vi "Autonomous Independent.vi"() -> ()   [LabVIEW 2013]
doc: "This VI is called when autonomous begins, and will automatically be terminated when autonomous ends. You can carry out timed or sensor driven robot movement independently without needing to return to the caller."
uses:
  Robot Global Data.vi
  <vilib>/Rock Robotics/WPI/Solenoid/Deprecated/WPI_SolenoidSetBool.vi
  <vilib>/Rock Robotics/WPI/Compressor/WPI_CompressorGetSetRefNum.vi
  <vilib>/Rock Robotics/WPI/RobotDrive/WPI_RobotDriveArcadeDrive_Standard(NoSaturation).vi
panel:
  in  "1 Ball Standard Auton Drive Length 2":dbl=11.0
  in  "final pickup delay":u32=1250
  in  "reload timeout 2":u32=4500
  in  "adjust out delay":u32=500
  in  "2 ball auton drive length":dbl=14.2
  in  "1st pickup delay 2":u32=500
  in  "Driving Shot Distance":dbl=10.0
  in  "Driving Shoot total distance":dbl=14.0
  in  "1 Ball Standard Auton Drive Length":dbl=11.0
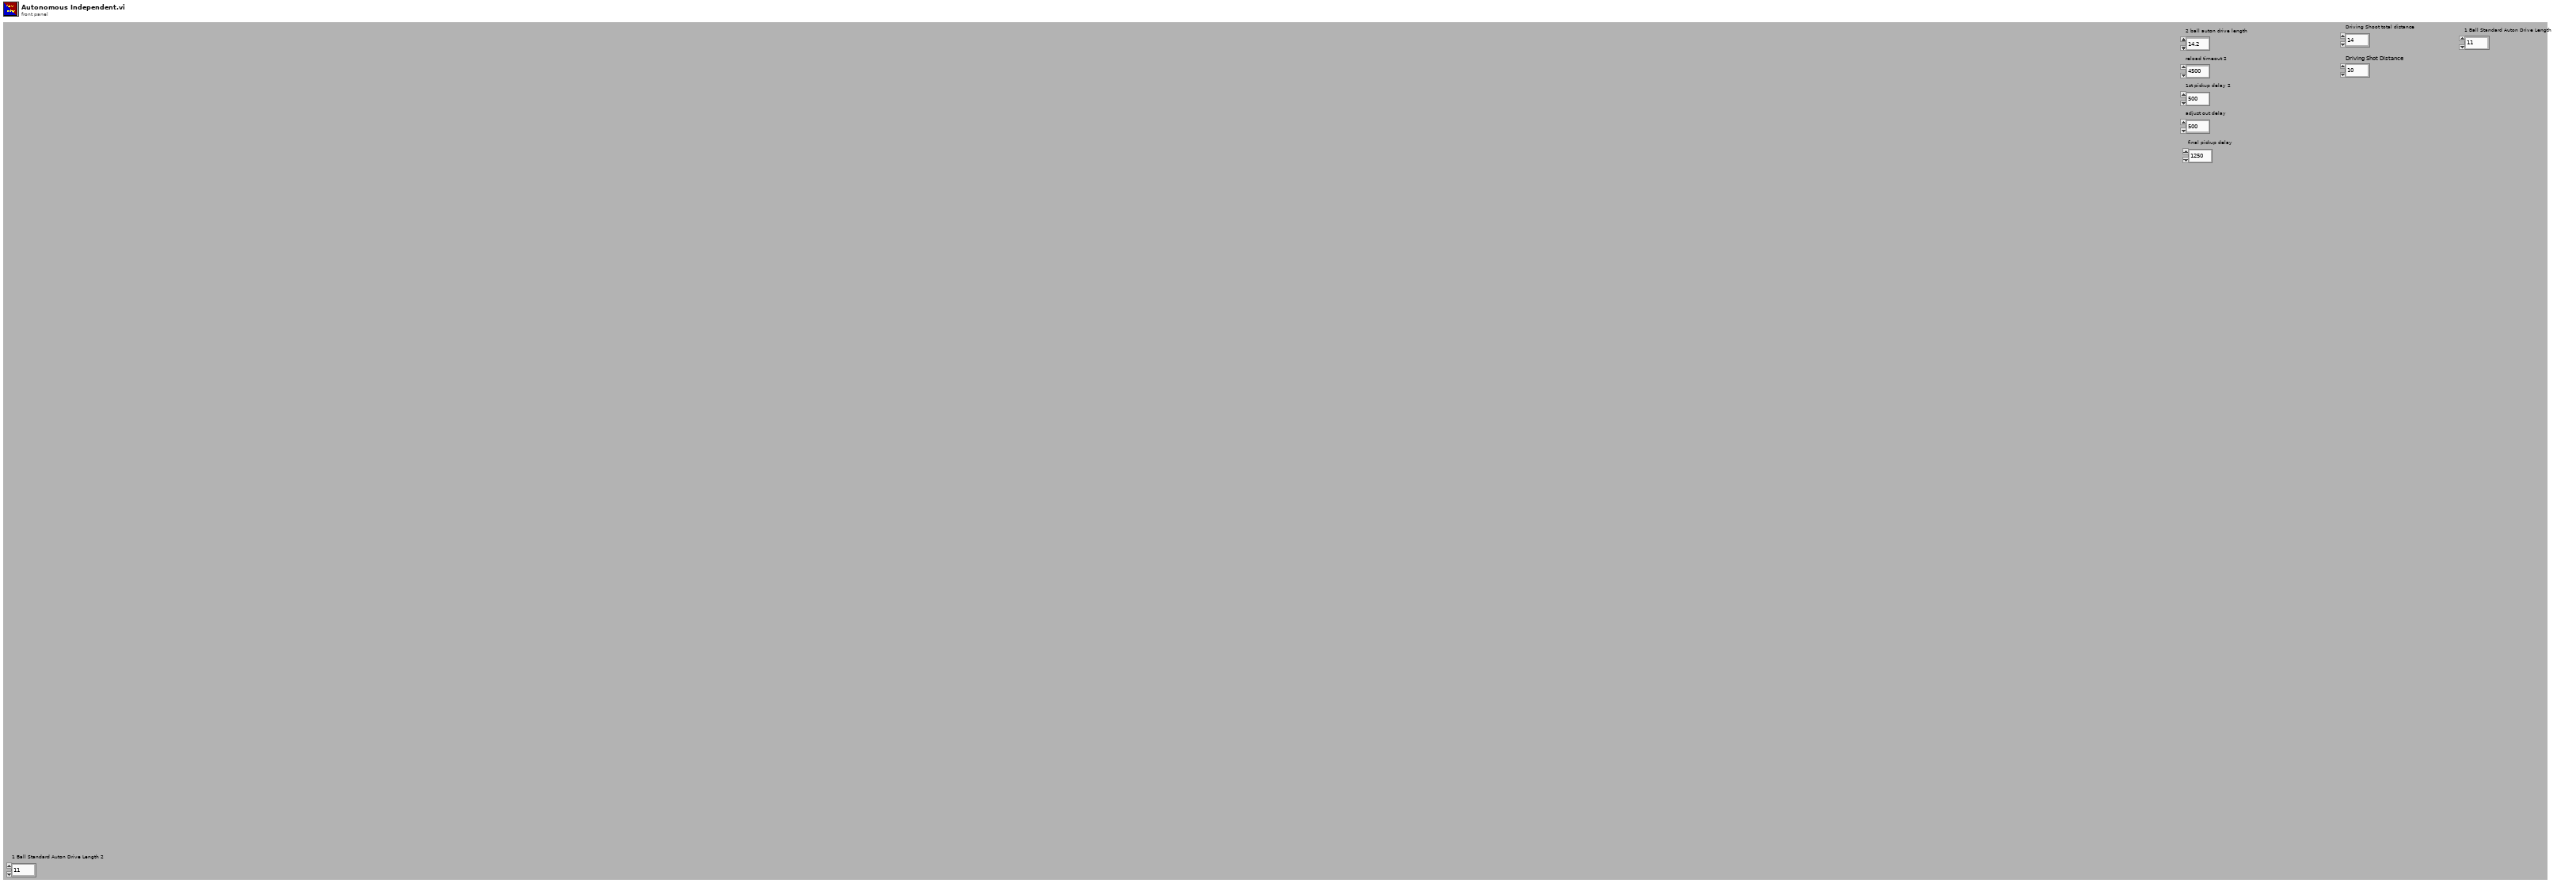
[diagram p1: front panel]
types:
  T1 = typedef "WPI_CompressorDevRef.ctl" = cluster{"DevStatus":errorcluster, "DigitalInputDevRef":T2, "RelayDevRef":T5}
  T2 = typedef "WPI_DigitalInputDevRef.ctl" = cluster{"DevStatus":errorcluster, "DIO Channel":T3, "Digital Module":T4}
  T3 = typedef "FPGA_DIOChannel.ctl" = enum8{"DIO 1", "DIO 2", "DIO 3", "DIO 4", "DIO 5", "DIO 6", "DIO 7", "DIO 8", "DIO 9", "DIO 10", "DIO 11", "DIO 12", "DIO 13", "DIO 14", "Invalid"}
  T4 = typedef "FPGA_TypedefDigitalModule.ctl" = enum16{"Digital Module 1", "Digital Module 2"}
  T5 = typedef "WPI_RelayDevRef.ctl" = cluster{"DevStatus":errorcluster, "Relay Channel":T6, "Digital Module":T4, "Relay Direction":T7}
  T6 = typedef "FPGA_DIORelayChannel.ctl" = enum8{"Relay 1", "Relay 2", "Relay 3", "Relay 4", "Relay 5", "Relay 6", "Relay 7", "Relay 8", "Invalid"}
  T7 = typedef "WPI_RelayDirection.ctl" = enum16{"Both directions", "Forward only", "Reverse only"}
  T8 = typedef "WPI_EncoderDevRef.ctl" = cluster{"DevStatus":errorcluster, "EncoderIndex":T9, "CounterIndex":T10, "DistancePerCount":dbl, "Decoding Type":T11}
  T9 = typedef "FPGA_EncoderIdx.ctl" = enum8{"Enc 0", "Enc 1", "Enc 2", "Enc 3", "Invalid"}
  T10 = typedef "FPGA_CounterCtrSystemIndex.ctl" = enum8{"Ctr 0", "Ctr 1", "Ctr 2", "Ctr 3", "Ctr 4", "Ctr 5", "Ctr 6", "Ctr 7", "Invalid"}
  T11 = typedef "WPI_EncoderType.ctl" = enum16{"1x", "2x", "4x"}
  T12 = typedef "WPI_SolenoidDevRef.ctl" = cluster{"DevStatus":errorcluster, "Solenoid Module":T13, "Forward Solenoid Channel":T14, "Reverse Solenoid Channel":T14}
  T13 = typedef "FPGA_TypedefSolenoidModule.ctl" = enum16{"Solenoid Module 1", "Solenoid Module 2"}
  T14 = typedef "WPI_SolenoidChannel.ctl" = enum8{"Solenoid 1", "Solenoid 2", "Solenoid 3", "Solenoid 4", "Solenoid 5", "Solenoid 6", "Solenoid 7", "Solenoid 8", "Invalid"}
  T15 = typedef "WPI_GyroDevRef.ctl" = cluster{"DevStatus":errorcluster, "Analog Module":T16, "Analog Channel":T17, "Offset":dbl, "Gain (VoltsPerDegree/Second)":dbl}
  T16 = typedef "FPGA_TypedefAnalogModule.ctl" = enum16{"Analog Module 1", "Analog Module 2"}
  T17 = typedef "FPGA_AIChannel.ctl" = enum8{"AI 1", "AI 2", "AI 3", "AI 4", "AI 5", "AI 6", "AI 7", "AI 8", "Invalid"}
  T18 = typedef "WPI_MotorControlDeviceRef.ctl" = cluster{"DeviceStatus":errorcluster, "Type":enum16{"PWM", "CAN"}, "PWM":cluster{"Digital Module":T4, "PWM Channel":T19, "DeadBand":T20}, "CAN":cluster{"Device Number":u8, "Control Mode":T21, "Semaphore":T22, "Max Vout":dbl}, "Invert":bool, "TransformRef":T23, "InvTransformRef":T23}
  T19 = typedef "FPGA_DIOPWMChannel.ctl" = enum8{"PWM 1", "PWM 2", "PWM 3", "PWM 4", "PWM 5", "PWM 6", "PWM 7", "PWM 8", "PWM 9", "PWM 10", "Invalid"}
  T20 = typedef "WPI_PWMDeadband.ctl" = cluster{"Name":string, "maxPositivePwm":i32, "minPositivePwm":i32, "centerPwm":i32, "maxNegativePwm":i32, "minNegativePwm":i32, "angularRange":u16}
  T21 = typedef "WPI_CANJaguar_ControlMode.ctl" = enum8{"Percent VBus", "Current", "Speed", "Position", "Voltage"}
  T22 = typedef "Semaphore RefNum" = refnum<k1>
  T23 = typedef "WPI_PWMTransform_ConPane.ctl" = refnum<vi>
  T24 = typedef "WPI_AnalogChannelDevRef.ctl" = cluster{"DevStatus":errorcluster, "Analog Module":T16, "Analog Channel":T17}
  T25 = typedef "WPI_RobotDriveDevRef.ctl" = cluster{"DevStatus":errorcluster, "Motors[]":T18[], "Square Inputs":bool, "Max Output":dbl, "Isochronous":bool}
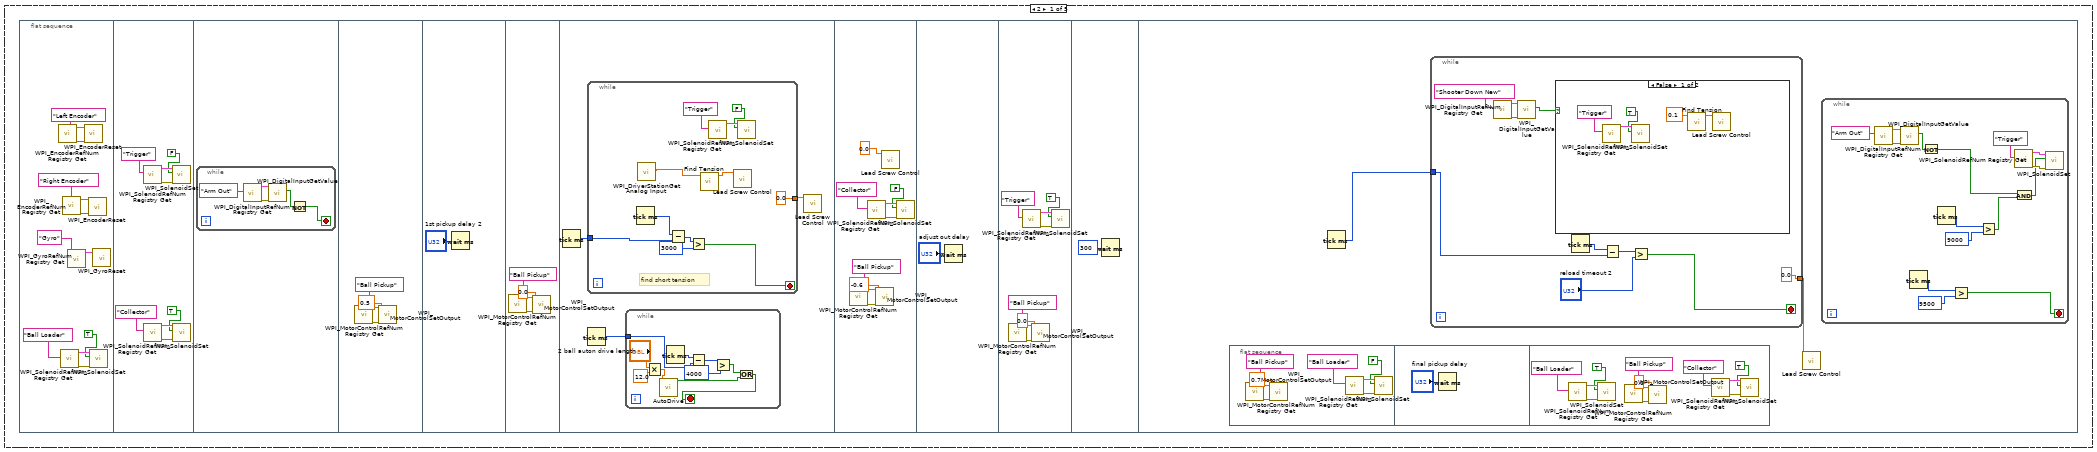
[diagram p2: hidden frame]
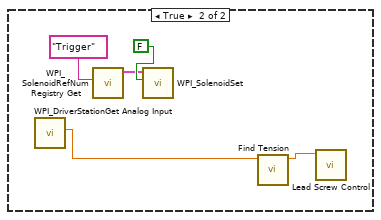
[diagram p3: hidden frame]
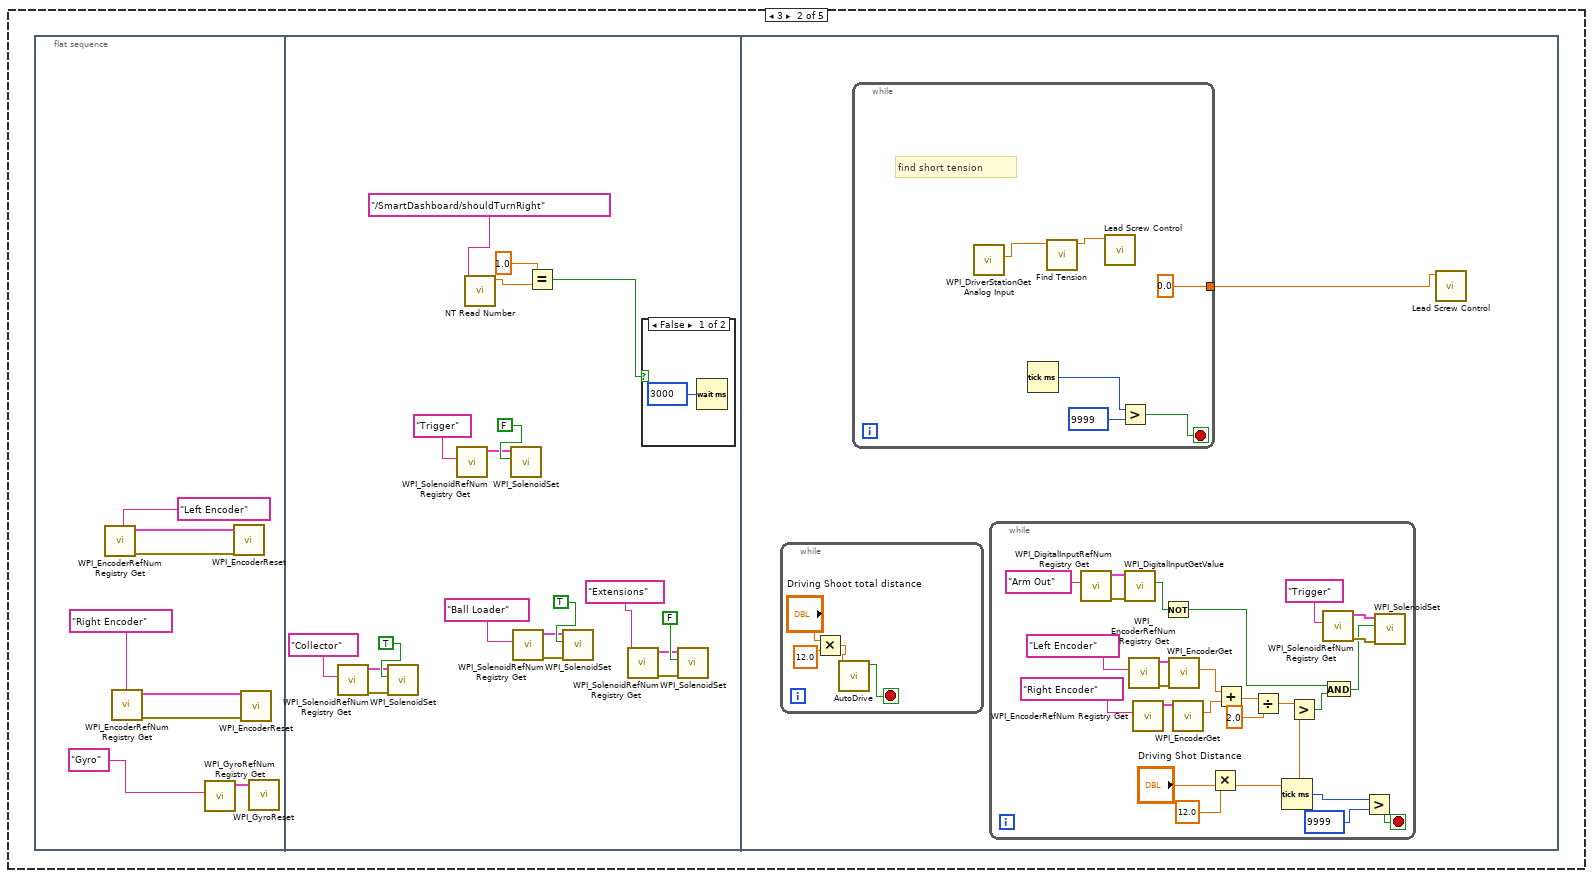
[diagram p4: hidden frame]
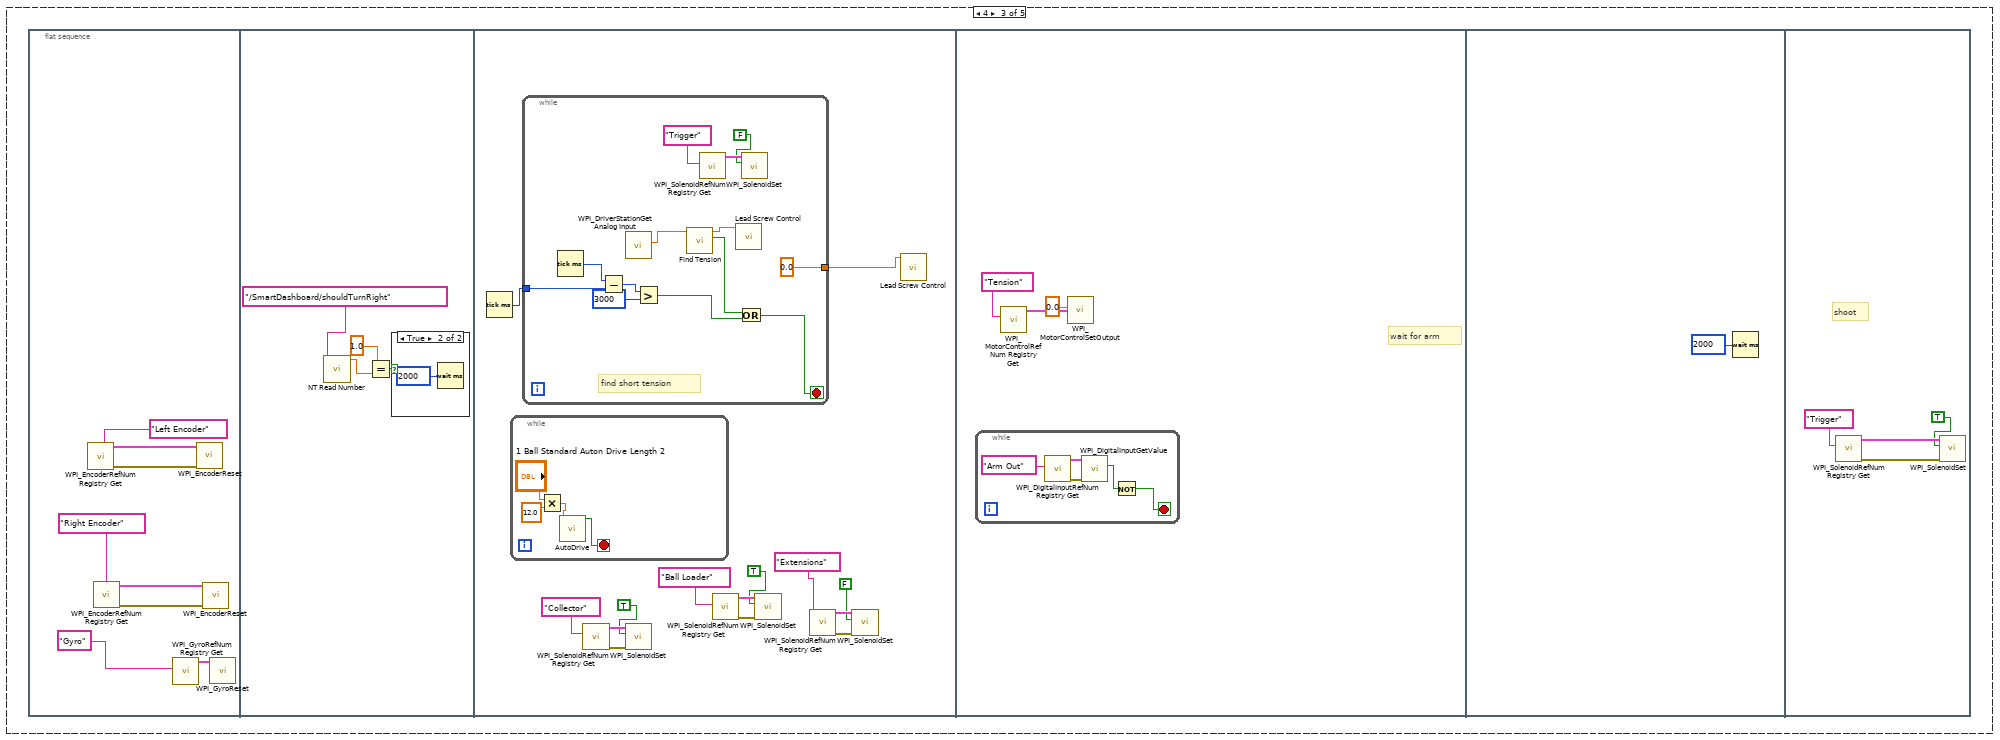
[diagram p6: hidden frame]
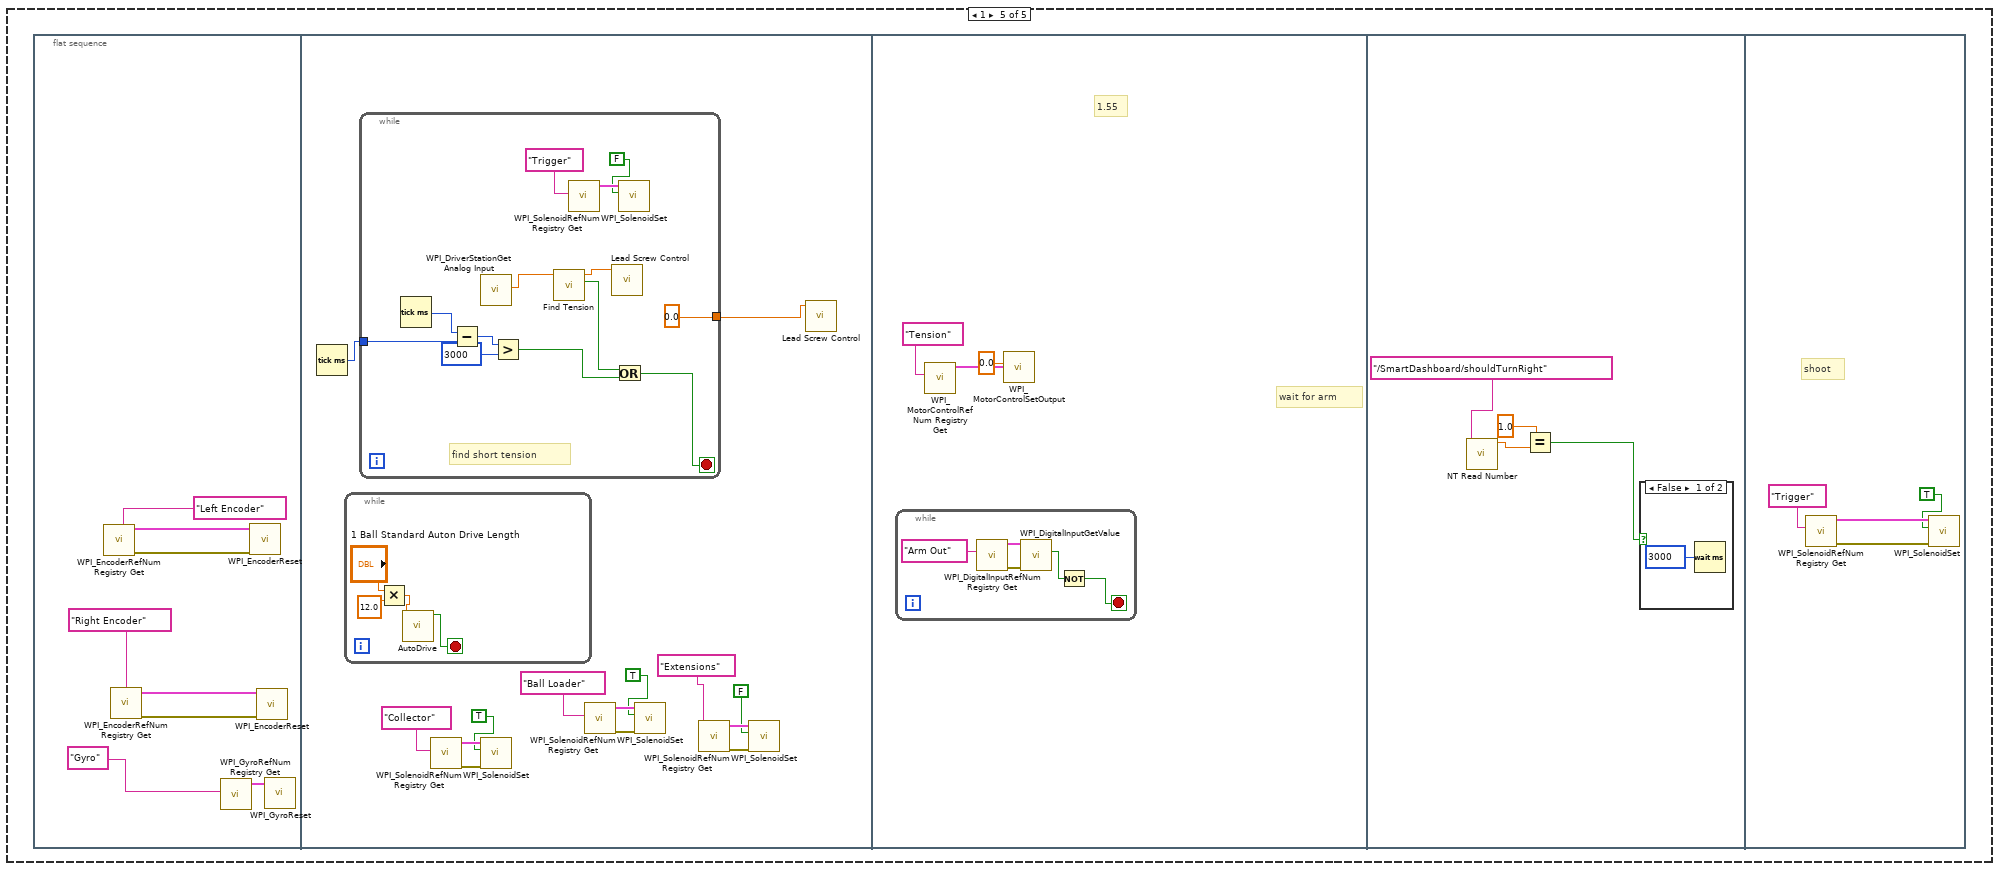
[diagram p8: hidden frame]
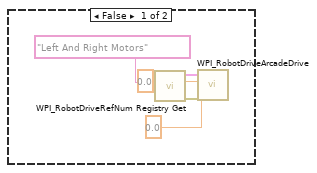
[diagram p10: hidden frame]
diagram:
  (unwired) "This code sets the toggle rate used by the Periodic Tasks VI.  For autonomous mode we slowly flash the USER1 LED on the cRIO.  Look at the Periodic Tasks VI to see how this global value is used."
  # "report tension"
  # "0 - nothing\n1 - standard 1-ball\n2 - 2 - ball auton \n3 - driving 1 ball"
  # "This gives you the four\nDriver Station sliders or\nanalog voltages"
  # "Every 20ms, report that we are running autonomous\ncode. Loop will abort the same time as the VI."
  n1 = call <vilib>:"WPI_DriverStationGet Analog Input.vi"() -> ("Analog 1 (V)"=w6:dbl)  [unwired: 11 out]
  n2 = call <vilib>:"WPI_CompressorRefNum Registry Get.vi"("refnum name"="Compressor") -> ("error out"=w3:errorcluster, "CompressorDevRef"=w2:T1)  [unwired: 9 in]
  n3 = Round To Nearest(number=w6) -> (nearest integer value=w5:dbl)
  n4 = call <vilib>:"WPI_CompressorStart.vi"("error in (no error)"=w3, "CompressorDevRef"=w2) -> ()  [unwired: 8 in, 2 out]
  n5 = case shown="0, Default" w5 {
    frame 2 {
      n6 = flat-sequence {
        frame #0 {
          n7 = call <vilib>:"WPI_EncoderRefNum Registry Get.vi"("refnum name"="Left Encoder") -> ("error out"=w18:errorcluster, "EncoderDevRef"=w17:T8)  [unwired: 9 in]
          n8 = call <vilib>:"WPI_SolenoidRefNum Registry Get.vi"("refnum name"="Ball Loader") -> ("error out"=w10:errorcluster, "SolenoidDevRef"=w9:T12)  [unwired: 9 in]
          n9 = call <vilib>:"WPI_EncoderRefNum Registry Get.vi"("refnum name"="Right Encoder") -> ("error out"=w16:errorcluster, "EncoderDevRef"=w15:T8)  [unwired: 9 in]
          n10 = call <vilib>:"WPI_GyroRefNum Registry Get.vi"("refnum name"="Gyro") -> ("GyroDevRef"=w11:T15)  [unwired: 9 in, 1 out]
          n11 = call <vilib>:"WPI_EncoderReset.vi"("error in (no error)"=w18, "EncoderDevRef"=w17) -> ()  [unwired: 8 in, 2 out]
          n12 = call <vilib>:"WPI_EncoderReset.vi"("error in (no error)"=w16, "EncoderDevRef"=w15) -> ()  [unwired: 8 in, 2 out]
          n13 = call-poly <vilib>:"WPI_SolenoidSet.vi"("error in (no error)"=w10, "Value"=TRUE, "SolenoidDevRef"=w9) -> ()  [unwired: 7 in, 2 out]
          n14 = call <vilib>:"WPI_GyroReset.vi"("GyroDevRef"=w11) -> ()  [unwired: 9 in, 2 out]
        }
        frame #1 {
          n15 = call <vilib>:"WPI_SolenoidRefNum Registry Get.vi"("refnum name"="Trigger") -> ("error out"=w26:errorcluster, "SolenoidDevRef"=w25:T12)  [unwired: 9 in]
          n16 = call <vilib>:"WPI_SolenoidRefNum Registry Get.vi"("refnum name"="Collector") -> ("error out"=w22:errorcluster, "SolenoidDevRef"=w21:T12)  [unwired: 9 in]
          n17 = call-poly <vilib>:"WPI_SolenoidSet.vi"("error in (no error)"=w26, "Value"=FALSE, "SolenoidDevRef"=w25) -> ()  [unwired: 7 in, 2 out]
          n18 = call-poly <vilib>:"WPI_SolenoidSet.vi"("error in (no error)"=w22, "Value"=TRUE, "SolenoidDevRef"=w21) -> ()  [unwired: 7 in, 2 out]
        }
        frame #2 {
          n19 = while {
            stop <- w28 stop-if-true
            n20 = call <vilib>:"WPI_DigitalInputRefNum Registry Get.vi"("refnum name"="Arm Out") -> ("error out"=w29:errorcluster, "DigitalInputDevRef"=w30:T2)  [unwired: 9 in]
            n21 = call <vilib>:"WPI_DigitalInputGetValue.vi"("error in (no error)"=w29, "DigitalInputDevRef"=w30) -> ("Value"=w27:bool)  [unwired: 7 in, 2 out]
            n22 = Not(x=w27) -> (.not. x?=w28:bool)
          }
        }
        frame #3 {
          n23 = call <vilib>:"WPI_MotorControlRefNum Registry Get.vi"("refnum name"="Ball Pickup") -> ("error out"=w34:errorcluster, "MotorControlDevRef"=w35:T18)  [unwired: 9 in]
          n24 = call <vilib>:"WPI_MotorControlSetOutput.vi"("error in (no error)"=w34, "Output"=0.5, "MotorControlDevRef"=w35) -> ()  [unwired: 6 in, 3 out]
        }
        frame #4 {
          n25 = Wait (ms)(milliseconds to wait="1st pickup delay 2") -> ()  [unwired: 1 out]
        }
        frame #5 {
          n26 = call <vilib>:"WPI_MotorControlRefNum Registry Get.vi"("refnum name"="Ball Pickup") -> ("error out"=w39:errorcluster, "MotorControlDevRef"=w40:T18)  [unwired: 9 in]
          n27 = call <vilib>:"WPI_MotorControlSetOutput.vi"("error in (no error)"=w39, "Output"=0.0, "MotorControlDevRef"=w40) -> ()  [unwired: 6 in, 3 out]
        }
        frame #6 {
          n28 = Tick Count (ms)() -> (millisecond timer value=w42:u32)
          n29 = while {
            tunnel: [0.0 ("Input Velocity")] -> w41
            tunnel: w42 -> [w58]
            stop <- w55 stop-if-true
            # "find short tension"
            n30 = Tick Count (ms)() -> (millisecond timer value=w59:u32)
            n31 = call <vilib>:"WPI_DriverStationGet Analog Input.vi"() -> ("Analog 2 (V)"=w54:dbl)  [unwired: 11 out]
            n32 = Subtract(x=w59, y=w58) -> (x-y=w57:u32)
            n33 = Greater?(x=w57, y=u32 3000) -> (0:w55:bool)
            n34 = call "Find Tension.vi"("Desired Tension"=w54) -> ("Motor Output"=w61:dbl)  [unwired: 9 in, 1 out]
            n35 = call <vilib>:"WPI_SolenoidRefNum Registry Get.vi"("refnum name"="Trigger") -> ("SolenoidDevRef"=w64:T12)  [unwired: 9 in, 1 out]
            n36 = call "Lead Screw Control.vi"("Input Velocity"=w61) -> ()  [unwired: 11 in]
            n37 = call-poly <vilib>:"WPI_SolenoidSet.vi"("Value"=FALSE, "SolenoidDevRef"=w64) -> ()  [unwired: 8 in, 2 out]
          }
          n38 = Tick Count (ms)() -> (millisecond timer value=w43:u32)
          n39 = while {
            tunnel: w43 -> [w49]
            stop <- w48 stop-if-true
            n40 = Multiply(x="2 ball auton drive length", y=12.0) -> (x*y=w53:dbl)
            n41 = call "AutoDrive.vi"("Target"=w53) -> ("Reached Target"=w47:bool)  [unwired: 10 in]
            n42 = Tick Count (ms)() -> (millisecond timer value=w50:u32)
            n43 = Subtract(x=w50, y=w49) -> (x-y=w45:u32)
            n44 = Greater?(x=w45, y=u32 4000) -> (0:w44:bool)
            n45 = Or(x=w44, y=w47) -> (x .or. y?=w48:bool)
          }
          n46 = call "Lead Screw Control.vi"("Input Velocity"=w41) -> ()  [unwired: 11 in]
        }
        frame #7 {
          n47 = call <vilib>:"WPI_MotorControlRefNum Registry Get.vi"("refnum name"="Ball Pickup") -> ("error out"=w67:errorcluster, "MotorControlDevRef"=w68:T18)  [unwired: 9 in]
          n48 = call <vilib>:"WPI_SolenoidRefNum Registry Get.vi"("refnum name"="Collector") -> ("error out"=w73:errorcluster, "SolenoidDevRef"=w72:T12)  [unwired: 9 in]
          n49 = call <vilib>:"WPI_MotorControlSetOutput.vi"("error in (no error)"=w67, "Output"=-0.6, "MotorControlDevRef"=w68) -> ()  [unwired: 6 in, 3 out]
          n50 = call "Lead Screw Control.vi"("Input Velocity"=0.0) -> ()  [unwired: 11 in]
          n51 = call-poly <vilib>:"WPI_SolenoidSet.vi"("error in (no error)"=w73, "Value"=FALSE, "SolenoidDevRef"=w72) -> ()  [unwired: 7 in, 2 out]
        }
        frame #8 {
          n52 = Wait (ms)(milliseconds to wait="adjust out delay") -> ()  [unwired: 1 out]
        }
        frame #9 {
          n53 = call <vilib>:"WPI_MotorControlRefNum Registry Get.vi"("refnum name"="Ball Pickup") -> ("error out"=w77:errorcluster, "MotorControlDevRef"=w78:T18)  [unwired: 9 in]
          n54 = call <vilib>:"WPI_SolenoidRefNum Registry Get.vi"("refnum name"="Trigger") -> ("error out"=w82:errorcluster, "SolenoidDevRef"=w81:T12)  [unwired: 9 in]
          n55 = call <vilib>:"WPI_MotorControlSetOutput.vi"("error in (no error)"=w77, "Output"=0.0, "MotorControlDevRef"=w78) -> ()  [unwired: 6 in, 3 out]
          n56 = call-poly <vilib>:"WPI_SolenoidSet.vi"("error in (no error)"=w82, "Value"=TRUE, "SolenoidDevRef"=w81) -> ()  [unwired: 7 in, 2 out]
        }
        frame #10 {
          n57 = Wait (ms)(milliseconds to wait=u32 300) -> ()  [unwired: 1 out]
        }
        frame #11 {
          n58 = flat-sequence {
            frame #0 {
              n59 = call <vilib>:"WPI_MotorControlRefNum Registry Get.vi"("refnum name"="Ball Pickup") -> ("error out"=w127:errorcluster, "MotorControlDevRef"=w128:T18)  [unwired: 9 in]
              n60 = call <vilib>:"WPI_MotorControlSetOutput.vi"("error in (no error)"=w127, "Output"=0.7, "MotorControlDevRef"=w128) -> ()  [unwired: 6 in, 3 out]
              n61 = call <vilib>:"WPI_SolenoidRefNum Registry Get.vi"("refnum name"="Ball Loader") -> ("error out"=w124:errorcluster, "SolenoidDevRef"=w123:T12)  [unwired: 9 in]
              n62 = call-poly <vilib>:"WPI_SolenoidSet.vi"("error in (no error)"=w124, "Value"=FALSE, "SolenoidDevRef"=w123) -> ()  [unwired: 7 in, 2 out]
            }
            frame #1 {
              n63 = Wait (ms)(milliseconds to wait="final pickup delay") -> ()  [unwired: 1 out]
            }
            frame #2 {
              n64 = call <vilib>:"WPI_SolenoidRefNum Registry Get.vi"("refnum name"="Ball Loader") -> ("error out"=w133:errorcluster, "SolenoidDevRef"=w132:T12)  [unwired: 9 in]
              n65 = call-poly <vilib>:"WPI_SolenoidSet.vi"("error in (no error)"=w133, "Value"=TRUE, "SolenoidDevRef"=w132) -> ()  [unwired: 7 in, 2 out]
              n66 = call <vilib>:"WPI_MotorControlRefNum Registry Get.vi"("refnum name"="Ball Pickup") -> ("error out"=w140:errorcluster, "MotorControlDevRef"=w141:T18)  [unwired: 9 in]
              n67 = call <vilib>:"WPI_MotorControlSetOutput.vi"("error in (no error)"=w140, "Output"=0.0, "MotorControlDevRef"=w141) -> ()  [unwired: 6 in, 3 out]
              n68 = call <vilib>:"WPI_SolenoidRefNum Registry Get.vi"("refnum name"="Collector") -> ("error out"=w137:errorcluster, "SolenoidDevRef"=w136:T12)  [unwired: 9 in]
              n69 = call-poly <vilib>:"WPI_SolenoidSet.vi"("error in (no error)"=w137, "Value"=TRUE, "SolenoidDevRef"=w136) -> ()  [unwired: 7 in, 2 out]
            }
          }
          n70 = Tick Count (ms)() -> (millisecond timer value=w85:u32)
          n71 = while {
            tunnel: w85 -> [w105]
            tunnel: [0.0] -> w84
            stop <- w101 stop-if-true
            n72 = call <vilib>:"WPI_DigitalInputRefNum Registry Get.vi"("refnum name"="Shooter Down New") -> ("error out"=w107:errorcluster, "DigitalInputDevRef"=w108:T2)  [unwired: 9 in]
            n73 = call <vilib>:"WPI_DigitalInputGetValue.vi"("error in (no error)"=w107, "DigitalInputDevRef"=w108) -> ("Value"=w110:bool)  [unwired: 7 in, 2 out]
            n74 = case shown="False" w110 {
              frame False {
                n75 = call <vilib>:"WPI_SolenoidRefNum Registry Get.vi"("refnum name"="Trigger") -> ("SolenoidDevRef"=w115:T12)  [unwired: 9 in, 1 out]
                n76 = call-poly <vilib>:"WPI_SolenoidSet.vi"("Value"=TRUE, "SolenoidDevRef"=w115) -> ()  [unwired: 8 in, 2 out]
                n77 = call "Find Tension.vi"("Desired Tension"=0.1) -> ("Motor Output"=w112:dbl)  [unwired: 9 in, 1 out]
                n78 = call "Lead Screw Control.vi"("Input Velocity"=w112) -> ()  [unwired: 11 in]
              }
              frame True {
                n79 = call <vilib>:"WPI_DriverStationGet Analog Input.vi"() -> ("Analog 2 (V)"=w116:dbl)  [unwired: 11 out]
                n80 = call <vilib>:"WPI_SolenoidRefNum Registry Get.vi"("refnum name"="Trigger") -> ("SolenoidDevRef"=w118:T12)  [unwired: 9 in, 1 out]
                n81 = call-poly <vilib>:"WPI_SolenoidSet.vi"("Value"=FALSE, "SolenoidDevRef"=w118) -> ()  [unwired: 8 in, 2 out]
                n82 = call "Find Tension.vi"("Desired Tension"=w116) -> ("Motor Output"=w117:dbl)  [unwired: 9 in, 1 out]
                n83 = call "Lead Screw Control.vi"("Input Velocity"=w117) -> ()  [unwired: 11 in]
              }
            }
            n84 = Tick Count (ms)() -> (millisecond timer value=w106:u32)
            n85 = Subtract(x=w106, y=w105) -> (x-y=w104:u32)
            n86 = Greater?(x=w104, y="reload timeout 2") -> (0:w101:bool)
          }
          n87 = call "Lead Screw Control.vi"("Input Velocity"=w84) -> ()  [unwired: 11 in]
          n88 = while {
            stop <- w86 stop-if-true
            n89 = call <vilib>:"WPI_DigitalInputRefNum Registry Get.vi"("refnum name"="Arm Out") -> ("error out"=w98:errorcluster, "DigitalInputDevRef"=w99:T2)  [unwired: 9 in]
            n90 = call <vilib>:"WPI_DigitalInputGetValue.vi"("error in (no error)"=w98, "DigitalInputDevRef"=w99) -> ("Value"=w97:bool)  [unwired: 7 in, 2 out]
            n91 = Tick Count (ms)() -> (millisecond timer value=w88:u32)
            n92 = Not(x=w97) -> (.not. x?=w93:bool)
            n93 = Tick Count (ms)() -> (millisecond timer value=w91:u32)
            n94 = Greater?(x=w88, y=u32 9500) -> (0:w86:bool)
            n95 = Greater?(x=w91, y=u32 9000) -> (0:w89:bool)
            n96 = call <vilib>:"WPI_SolenoidRefNum Registry Get.vi"("refnum name"="Trigger") -> ("error out"=w94:errorcluster, "SolenoidDevRef"=w95:T12)  [unwired: 9 in]
            n97 = And(x=w93, y=w89) -> (x .and. y?=w92:bool)
            n98 = call-poly <vilib>:"WPI_SolenoidSet.vi"("error in (no error)"=w94, "Value"=w92, "SolenoidDevRef"=w95) -> ()  [unwired: 7 in, 2 out]
          }
        }
      }
    }
    frame 3 {
      n99 = flat-sequence {
        frame #0 {
          n100 = call <vilib>:"WPI_EncoderRefNum Registry Get.vi"("refnum name"="Left Encoder") -> ("error out"=w149:errorcluster, "EncoderDevRef"=w148:T8)  [unwired: 9 in]
          n101 = call <vilib>:"WPI_EncoderRefNum Registry Get.vi"("refnum name"="Right Encoder") -> ("error out"=w147:errorcluster, "EncoderDevRef"=w146:T8)  [unwired: 9 in]
          n102 = call <vilib>:"WPI_GyroRefNum Registry Get.vi"("refnum name"="Gyro") -> ("GyroDevRef"=w142:T15)  [unwired: 9 in, 1 out]
          n103 = call <vilib>:"WPI_EncoderReset.vi"("error in (no error)"=w149, "EncoderDevRef"=w148) -> ()  [unwired: 8 in, 2 out]
          n104 = call <vilib>:"WPI_EncoderReset.vi"("error in (no error)"=w147, "EncoderDevRef"=w146) -> ()  [unwired: 8 in, 2 out]
          n105 = call <vilib>:"WPI_GyroReset.vi"("GyroDevRef"=w142) -> ()  [unwired: 9 in, 2 out]
        }
        frame #1 {
          n106 = call <vilib>:"WPI_SolenoidRefNum Registry Get.vi"("refnum name"="Collector") -> ("error out"=w161:errorcluster, "SolenoidDevRef"=w162:T12)  [unwired: 9 in]
          n107 = call-poly <vilib>:"WPI_SolenoidSet.vi"("error in (no error)"=w161, "Value"=TRUE, "SolenoidDevRef"=w162) -> ()  [unwired: 7 in, 2 out]
          n108 = call <vilib>:"WPI_SolenoidRefNum Registry Get.vi"("refnum name"="Trigger") -> ("SolenoidDevRef"=w150:T12)  [unwired: 9 in, 1 out]
          n109 = call <vilib>:"NT Read Number.vi"("Name"="/SmartDashboard/shouldTurnRight") -> ("Numeric"=w168:dbl)  [unwired: 9 in, 1 out]
          n110 = call-poly <vilib>:"WPI_SolenoidSet.vi"("Value"=FALSE, "SolenoidDevRef"=w150) -> ()  [unwired: 8 in, 2 out]
          n111 = call <vilib>:"WPI_SolenoidRefNum Registry Get.vi"("refnum name"="Ball Loader") -> ("error out"=w153:errorcluster, "SolenoidDevRef"=w154:T12)  [unwired: 9 in]
          n112 = Equal?(x=1.0, y=w168) -> (x = y?=w165:bool)
          n113 = call-poly <vilib>:"WPI_SolenoidSet.vi"("error in (no error)"=w153, "Value"=TRUE, "SolenoidDevRef"=w154) -> ()  [unwired: 7 in, 2 out]
          n114 = call <vilib>:"WPI_SolenoidRefNum Registry Get.vi"("refnum name"="Extensions") -> ("error out"=w160:errorcluster, "SolenoidDevRef"=w157:T12)  [unwired: 9 in]
          n115 = case shown="False" w165 {
            frame False {
              n116 = Wait (ms)(milliseconds to wait=u32 3000) -> ()  [unwired: 1 out]
            }
            frame True {
            }
          }
          n117 = call-poly <vilib>:"WPI_SolenoidSet.vi"("error in (no error)"=w160, "Value"=FALSE, "SolenoidDevRef"=w157) -> ()  [unwired: 7 in, 2 out]
        }
        frame #2 {
          n118 = while {
            stop <- w206 stop-if-true
            n119 = Multiply(x="Driving Shoot total distance", y=12.0) -> (x*y=w205:dbl)
            n120 = call "AutoDrive.vi"("Target"=w205) -> ("Reached Target"=w206:bool)  [unwired: 10 in]
          }
          n121 = while {
            tunnel: [0.0 ("Input Velocity")] -> w170
            stop <- w171 stop-if-true
            # "find short tension"
            n122 = call <vilib>:"WPI_DriverStationGet Analog Input.vi"() -> ("Analog 2 (V)"=w173:dbl)  [unwired: 11 out]
            n123 = Tick Count (ms)() -> (millisecond timer value=w172:u32)
            n124 = call "Find Tension.vi"("Desired Tension"=w173) -> ("Motor Output"=w176:dbl)  [unwired: 9 in, 1 out]
            n125 = call "Lead Screw Control.vi"("Input Velocity"=w176) -> ()  [unwired: 11 in]
            n126 = Greater?(x=w172, y=u32 9999) -> (0:w171:bool)
          }
          n127 = while {
            stop <- w179 stop-if-true
            n128 = call <vilib>:"WPI_DigitalInputRefNum Registry Get.vi"("refnum name"="Arm Out") -> ("error out"=w200:errorcluster, "DigitalInputDevRef"=w201:T2)  [unwired: 9 in]
            n129 = call <vilib>:"WPI_DigitalInputGetValue.vi"("error in (no error)"=w200, "DigitalInputDevRef"=w201) -> ("Value"=w199:bool)  [unwired: 7 in, 2 out]
            n130 = call <vilib>:"WPI_EncoderRefNum Registry Get.vi"("refnum name"="Left Encoder") -> ("error out"=w195:errorcluster, "EncoderDevRef"=w194:T8)  [unwired: 9 in]
            n131 = call <vilib>:"WPI_EncoderRefNum Registry Get.vi"("refnum name"="Right Encoder") -> ("EncoderDevRef"=w192:T8)  [unwired: 9 in, 1 out]
            n132 = Not(x=w199) -> (.not. x?=w183:bool)
            n133 = call <vilib>:"WPI_EncoderGet.vi"("error in (no error)"=w195, "EncoderDevRef"=w194) -> ("Distance"=w189:dbl)  [unwired: 4 in, 5 out]
            n134 = call <vilib>:"WPI_EncoderGet.vi"("EncoderDevRef"=w192) -> ("Distance"=w190:dbl)  [unwired: 5 in, 5 out]
            n135 = Multiply(x=12.0, y="Driving Shot Distance") -> (x*y=w178:dbl)
            n136 = Add(x=w189, y=w190) -> (x+y=w188:dbl)
            n137 = Divide(x=w188, y=2.0) -> (x/y=w186:dbl)
            n138 = Tick Count (ms)() -> (millisecond timer value=w181:u32)
            n139 = Greater?(x=w186, y=w178) -> (0:w184:bool)
            n140 = call <vilib>:"WPI_SolenoidRefNum Registry Get.vi"("refnum name"="Trigger") -> ("error out"=w196:errorcluster, "SolenoidDevRef"=w197:T12)  [unwired: 9 in]
            n141 = And(x=w183, y=w184) -> (x .and. y?=w182:bool)
            n142 = Greater?(x=w181, y=u32 9999) -> (0:w179:bool)
            n143 = call-poly <vilib>:"WPI_SolenoidSet.vi"("error in (no error)"=w196, "Value"=w182, "SolenoidDevRef"=w197) -> ()  [unwired: 7 in, 2 out]
          }
          n144 = call "Lead Screw Control.vi"("Input Velocity"=w170) -> ()  [unwired: 11 in]
        }
      }
    }
    frame 4 {
      n145 = flat-sequence {
        frame #0 {
          n146 = call <vilib>:"WPI_EncoderRefNum Registry Get.vi"("refnum name"="Left Encoder") -> ("error out"=w214:errorcluster, "EncoderDevRef"=w213:T8)  [unwired: 9 in]
          n147 = call <vilib>:"WPI_EncoderRefNum Registry Get.vi"("refnum name"="Right Encoder") -> ("error out"=w212:errorcluster, "EncoderDevRef"=w211:T8)  [unwired: 9 in]
          n148 = call <vilib>:"WPI_GyroRefNum Registry Get.vi"("refnum name"="Gyro") -> ("GyroDevRef"=w207:T15)  [unwired: 9 in, 1 out]
          n149 = call <vilib>:"WPI_EncoderReset.vi"("error in (no error)"=w214, "EncoderDevRef"=w213) -> ()  [unwired: 8 in, 2 out]
          n150 = call <vilib>:"WPI_EncoderReset.vi"("error in (no error)"=w212, "EncoderDevRef"=w211) -> ()  [unwired: 8 in, 2 out]
          n151 = call <vilib>:"WPI_GyroReset.vi"("GyroDevRef"=w207) -> ()  [unwired: 9 in, 2 out]
        }
        frame #1 {
          n152 = call <vilib>:"NT Read Number.vi"("Name"="/SmartDashboard/shouldTurnRight") -> ("Numeric"=w218:dbl)  [unwired: 9 in, 1 out]
          n153 = Equal?(x=1.0, y=w218) -> (x = y?=w215:bool)
          n154 = case shown="True" w215 {
            frame False {
            }
            frame True {
              n155 = Wait (ms)(milliseconds to wait=u32 2000) -> ()  [unwired: 1 out]
            }
          }
        }
        frame #2 {
          n156 = Tick Count (ms)() -> (millisecond timer value=w221:u32)
          n157 = while {
            stop <- w237 stop-if-true
            n158 = Multiply(x="1 Ball Standard Auton Drive Length 2", y=12.0) -> (x*y=w236:dbl)
            n159 = call "AutoDrive.vi"("Target"=w236) -> ("Reached Target"=w237:bool)  [unwired: 10 in]
          }
          n160 = while {
            tunnel: w221 -> [w245]
            tunnel: [0.0 ("Input Velocity")] -> w220
            stop <- w240 stop-if-true
            # "find short tension"
            n161 = Tick Count (ms)() -> (millisecond timer value=w246:u32)
            n162 = Subtract(x=w246, y=w245) -> (x-y=w244:u32)
            n163 = call <vilib>:"WPI_DriverStationGet Analog Input.vi"() -> ("Analog 2 (V)"=w238:dbl)  [unwired: 11 out]
            n164 = Greater?(x=w244, y=u32 3000) -> (0:w242:bool)
            n165 = call "Find Tension.vi"("Desired Tension"=w238) -> ("At Tension?"=w241:bool, "Motor Output"=w247:dbl)  [unwired: 9 in]
            n166 = call <vilib>:"WPI_SolenoidRefNum Registry Get.vi"("refnum name"="Trigger") -> ("SolenoidDevRef"=w250:T12)  [unwired: 9 in, 1 out]
            n167 = call "Lead Screw Control.vi"("Input Velocity"=w247) -> ()  [unwired: 11 in]
            n168 = Or(x=w241, y=w242) -> (x .or. y?=w240:bool)
            n169 = call-poly <vilib>:"WPI_SolenoidSet.vi"("Value"=FALSE, "SolenoidDevRef"=w250) -> ()  [unwired: 8 in, 2 out]
          }
          n170 = call <vilib>:"WPI_SolenoidRefNum Registry Get.vi"("refnum name"="Collector") -> ("error out"=w225:errorcluster, "SolenoidDevRef"=w224:T12)  [unwired: 9 in]
          n171 = call-poly <vilib>:"WPI_SolenoidSet.vi"("error in (no error)"=w225, "Value"=TRUE, "SolenoidDevRef"=w224) -> ()  [unwired: 7 in, 2 out]
          n172 = call <vilib>:"WPI_SolenoidRefNum Registry Get.vi"("refnum name"="Ball Loader") -> ("error out"=w233:errorcluster, "SolenoidDevRef"=w232:T12)  [unwired: 9 in]
          n173 = call-poly <vilib>:"WPI_SolenoidSet.vi"("error in (no error)"=w233, "Value"=TRUE, "SolenoidDevRef"=w232) -> ()  [unwired: 7 in, 2 out]
          n174 = call <vilib>:"WPI_SolenoidRefNum Registry Get.vi"("refnum name"="Extensions") -> ("error out"=w226:errorcluster, "SolenoidDevRef"=w229:T12)  [unwired: 9 in]
          n175 = call-poly <vilib>:"WPI_SolenoidSet.vi"("error in (no error)"=w226, "Value"=FALSE, "SolenoidDevRef"=w229) -> ()  [unwired: 7 in, 2 out]
          n176 = call "Lead Screw Control.vi"("Input Velocity"=w220) -> ()  [unwired: 11 in]
        }
        frame #3 {
          # "wait for arm"
          n177 = while {
            stop <- w255 stop-if-true
            n178 = call <vilib>:"WPI_DigitalInputRefNum Registry Get.vi"("refnum name"="Arm Out") -> ("error out"=w256:errorcluster, "DigitalInputDevRef"=w257:T2)  [unwired: 9 in]
            n179 = call <vilib>:"WPI_DigitalInputGetValue.vi"("error in (no error)"=w256, "DigitalInputDevRef"=w257) -> ("Value"=w254:bool)  [unwired: 7 in, 2 out]
            n180 = Not(x=w254) -> (.not. x?=w255:bool)
          }
          n181 = call <vilib>:"WPI_MotorControlRefNum Registry Get.vi"("refnum name"="Tension") -> ("MotorControlDevRef"=w253:T18)  [unwired: 9 in, 1 out]
          n182 = call <vilib>:"WPI_MotorControlSetOutput.vi"("Output"=0.0, "MotorControlDevRef"=w253) -> ()  [unwired: 7 in, 3 out]
        }
        frame #4 {
          n183 = Wait (ms)(milliseconds to wait=u32 2000) -> ()  [unwired: 1 out]
        }
        frame #5 {
          # "shoot"
          n184 = call <vilib>:"WPI_SolenoidRefNum Registry Get.vi"("refnum name"="Trigger") -> ("error out"=w263:errorcluster, "SolenoidDevRef"=w262:T12)  [unwired: 9 in]
          n185 = call-poly <vilib>:"WPI_SolenoidSet.vi"("error in (no error)"=w263, "Value"=TRUE, "SolenoidDevRef"=w262) -> ()  [unwired: 7 in, 2 out]
        }
      }
    }
    frame 0, Default {
      # "nothing"
      n186 = flat-sequence {
        frame #0 {
          n187 = call <vilib>:"WPI_EncoderRefNum Registry Get.vi"("refnum name"="Left Encoder") -> ("error out"=w271:errorcluster, "EncoderDevRef"=w270:T8)  [unwired: 9 in]
          n188 = call <vilib>:"WPI_EncoderRefNum Registry Get.vi"("refnum name"="Right Encoder") -> ("error out"=w269:errorcluster, "EncoderDevRef"=w268:T8)  [unwired: 9 in]
          n189 = call <vilib>:"WPI_GyroRefNum Registry Get.vi"("refnum name"="Gyro") -> ("GyroDevRef"=w264:T15)  [unwired: 9 in, 1 out]
          n190 = call <vilib>:"WPI_EncoderReset.vi"("error in (no error)"=w271, "EncoderDevRef"=w270) -> ()  [unwired: 8 in, 2 out]
          n191 = call <vilib>:"WPI_EncoderReset.vi"("error in (no error)"=w269, "EncoderDevRef"=w268) -> ()  [unwired: 8 in, 2 out]
          n192 = call <vilib>:"WPI_GyroReset.vi"("GyroDevRef"=w264) -> ()  [unwired: 9 in, 2 out]
        }
        frame #1 {
          n193 = while {
            stop <- w272 stop-if-true
            n194 = Multiply(x=10.0, y=12.0) -> (x*y=w275:dbl)
            n195 = call "AutoDrive.vi"("Target"=w275) -> ("Reached Target"=w272:bool)  [unwired: 10 in]
          }
        }
      }
    }
    frame 1 {
      n196 = flat-sequence {
        frame #0 {
          n197 = call <vilib>:"WPI_EncoderRefNum Registry Get.vi"("refnum name"="Left Encoder") -> ("error out"=w283:errorcluster, "EncoderDevRef"=w282:T8)  [unwired: 9 in]
          n198 = call <vilib>:"WPI_EncoderRefNum Registry Get.vi"("refnum name"="Right Encoder") -> ("error out"=w281:errorcluster, "EncoderDevRef"=w280:T8)  [unwired: 9 in]
          n199 = call <vilib>:"WPI_GyroRefNum Registry Get.vi"("refnum name"="Gyro") -> ("GyroDevRef"=w276:T15)  [unwired: 9 in, 1 out]
          n200 = call <vilib>:"WPI_EncoderReset.vi"("error in (no error)"=w283, "EncoderDevRef"=w282) -> ()  [unwired: 8 in, 2 out]
          n201 = call <vilib>:"WPI_EncoderReset.vi"("error in (no error)"=w281, "EncoderDevRef"=w280) -> ()  [unwired: 8 in, 2 out]
          n202 = call <vilib>:"WPI_GyroReset.vi"("GyroDevRef"=w276) -> ()  [unwired: 9 in, 2 out]
        }
        frame #1 {
          n203 = Tick Count (ms)() -> (millisecond timer value=w285:u32)
          n204 = while {
            stop <- w301 stop-if-true
            n205 = Multiply(x="1 Ball Standard Auton Drive Length", y=12.0) -> (x*y=w300:dbl)
            n206 = call "AutoDrive.vi"("Target"=w300) -> ("Reached Target"=w301:bool)  [unwired: 10 in]
          }
          n207 = while {
            tunnel: w285 -> [w309]
            tunnel: [0.0 ("Input Velocity")] -> w284
            stop <- w304 stop-if-true
            # "find short tension"
            n208 = Tick Count (ms)() -> (millisecond timer value=w310:u32)
            n209 = Subtract(x=w310, y=w309) -> (x-y=w308:u32)
            n210 = call <vilib>:"WPI_DriverStationGet Analog Input.vi"() -> ("Analog 2 (V)"=w302:dbl)  [unwired: 11 out]
            n211 = Greater?(x=w308, y=u32 3000) -> (0:w306:bool)
            n212 = call "Find Tension.vi"("Desired Tension"=w302) -> ("At Tension?"=w305:bool, "Motor Output"=w311:dbl)  [unwired: 9 in]
            n213 = call <vilib>:"WPI_SolenoidRefNum Registry Get.vi"("refnum name"="Trigger") -> ("SolenoidDevRef"=w314:T12)  [unwired: 9 in, 1 out]
            n214 = call "Lead Screw Control.vi"("Input Velocity"=w311) -> ()  [unwired: 11 in]
            n215 = Or(x=w305, y=w306) -> (x .or. y?=w304:bool)
            n216 = call-poly <vilib>:"WPI_SolenoidSet.vi"("Value"=FALSE, "SolenoidDevRef"=w314) -> ()  [unwired: 8 in, 2 out]
          }
          n217 = call <vilib>:"WPI_SolenoidRefNum Registry Get.vi"("refnum name"="Collector") -> ("error out"=w289:errorcluster, "SolenoidDevRef"=w288:T12)  [unwired: 9 in]
          n218 = call-poly <vilib>:"WPI_SolenoidSet.vi"("error in (no error)"=w289, "Value"=TRUE, "SolenoidDevRef"=w288) -> ()  [unwired: 7 in, 2 out]
          n219 = call <vilib>:"WPI_SolenoidRefNum Registry Get.vi"("refnum name"="Ball Loader") -> ("error out"=w297:errorcluster, "SolenoidDevRef"=w296:T12)  [unwired: 9 in]
          n220 = call-poly <vilib>:"WPI_SolenoidSet.vi"("error in (no error)"=w297, "Value"=TRUE, "SolenoidDevRef"=w296) -> ()  [unwired: 7 in, 2 out]
          n221 = call <vilib>:"WPI_SolenoidRefNum Registry Get.vi"("refnum name"="Extensions") -> ("error out"=w290:errorcluster, "SolenoidDevRef"=w293:T12)  [unwired: 9 in]
          n222 = call-poly <vilib>:"WPI_SolenoidSet.vi"("error in (no error)"=w290, "Value"=FALSE, "SolenoidDevRef"=w293) -> ()  [unwired: 7 in, 2 out]
          n223 = call "Lead Screw Control.vi"("Input Velocity"=w284) -> ()  [unwired: 11 in]
        }
        frame #2 {
          # "1.55"
          # "wait for arm"
          n224 = while {
            stop <- w319 stop-if-true
            n225 = call <vilib>:"WPI_DigitalInputRefNum Registry Get.vi"("refnum name"="Arm Out") -> ("error out"=w320:errorcluster, "DigitalInputDevRef"=w321:T2)  [unwired: 9 in]
            n226 = call <vilib>:"WPI_DigitalInputGetValue.vi"("error in (no error)"=w320, "DigitalInputDevRef"=w321) -> ("Value"=w318:bool)  [unwired: 7 in, 2 out]
            n227 = Not(x=w318) -> (.not. x?=w319:bool)
          }
          n228 = call <vilib>:"WPI_MotorControlRefNum Registry Get.vi"("refnum name"="Tension") -> ("MotorControlDevRef"=w317:T18)  [unwired: 9 in, 1 out]
          n229 = call <vilib>:"WPI_MotorControlSetOutput.vi"("Output"=0.0, "MotorControlDevRef"=w317) -> ()  [unwired: 7 in, 3 out]
        }
        frame #3 {
          n230 = call <vilib>:"NT Read Number.vi"("Name"="/SmartDashboard/shouldTurnRight") -> ("Numeric"=w326:dbl)  [unwired: 9 in, 1 out]
          n231 = Equal?(x=1.0, y=w326) -> (x = y?=w323:bool)
          n232 = case shown="False" w323 {
            frame False {
              n233 = Wait (ms)(milliseconds to wait=u32 3000) -> ()  [unwired: 1 out]
            }
            frame True {
            }
          }
        }
        frame #4 {
          # "shoot"
          n234 = call <vilib>:"WPI_SolenoidRefNum Registry Get.vi"("refnum name"="Trigger") -> ("error out"=w331:errorcluster, "SolenoidDevRef"=w330:T12)  [unwired: 9 in]
          n235 = call-poly <vilib>:"WPI_SolenoidSet.vi"("error in (no error)"=w331, "Value"=TRUE, "SolenoidDevRef"=w330) -> ()  [unwired: 7 in, 2 out]
        }
      }
    }
  }
  n236 = while {
    stop <- w332 stop-if-true
    n237 = Tick Count (ms)() -> (millisecond timer value=w334:u32)
    n238 = call <vilib>:"WPI_AnalogChannelRefNum Registry Get.vi"("refnum name"="Tension Potentiometer") -> ("error out"=w341:errorcluster, "AIDeviceRef"=w340:T24)  [unwired: 9 in]
    n239 = Greater?(x=w334, y=u32 9000) -> (0:w332:bool)
    n240 = call <vilib>:"WPI_AnalogChannelGetVoltage.vi"("error in (no error)"=w341, "AIDeviceRef"=w340) -> ("Voltage"=w337:dbl)  [unwired: 7 in, 2 out]
    n241 = Subtract(x=5.0, y=w337) -> (x-y=w335:dbl)
    n242 = call <vilib>:"SD Write Number.vi"("Numeric"=w335, "Name"="Tension Potentiometer") -> ()  [unwired: 8 in, 2 out]
  }
  n243 = while {
    stop <- FALSE stop-if-true
    n244 = call <vilib>:"WPI_DriverStationReport Robot Code State.vi"("Autonomous"=TRUE) -> ()  [unwired: 10 in, 1 out]
    n245 = Wait (ms)(milliseconds to wait=u32 20) -> ()  [unwired: 1 out]
  }
  n246 = global write "Robot Global Data.vi" "LED toggle rate (ms)"(u32 500 ("LED ms toggle rate")) -> ()
  n247 = disable-structure shown="Disabled" {
    frame Disabled {
      n248 = while {
        stop <- w345 stop-if-true
        n249 = Tick Count (ms)() -> (millisecond timer value=w347:u32)
        n250 = call-poly <vilib>:"NT Read Value.vi"("Name"="/SmartDashboard/BLOB_COUNT") -> ("Numeric"=w351:dbl)  [unwired: 9 in, 1 out]
        n251 = Add(x=u32 15000) -> (x+y=w346:u32)  [unwired: 1 in]
        n252 = Equal?(x=w351, y=1.0) -> (x = y?=w349:bool)
        n253 = case shown="True" w349 {
          frame False {
            n254 = call <vilib>:"WPI_RobotDriveRefNum Registry Get.vi"("refnum name"="Left And Right Motors") -> ("error out"=w358:errorcluster, "RobotDriveDevRef"=w357:T25)  [unwired: 9 in]
            n255 = call-poly <vilib>:"WPI_RobotDriveArcadeDrive.vi"("error in (no error)"=w358, "Y axis value"=0.0, "X axis value"=0.0, "RobotDriveDevRef"=w357) -> ()  [unwired: 5 in, 3 out]
          }
          frame True {
            n256 = call-poly <vilib>:"NT Read Value.vi"("Name"="/SmartDashboard/COG_X") -> ("Numeric"=w366:dbl)  [unwired: 9 in, 1 out]
            n257 = Subtract(x=w366, y=240.0) -> (x-y=w364:dbl)
            n258 = Divide(x=w364, y=100.0) -> (x/y=w362:dbl)
            n259 = Absolute Value(x=w362) -> (abs(x)=w361:dbl)
            n260 = Y-th Root of X(1:w361, 2:3.0 ("y")) -> (0:w359:dbl)
            n261 = call <vilib>:"WPI_RobotDriveRefNum Registry Get.vi"("refnum name"="Left And Right Motors") -> ("error out"=w370:errorcluster, "RobotDriveDevRef"=w369:T25)  [unwired: 9 in]
            n262 = call-poly <vilib>:"WPI_RobotDriveArcadeDrive.vi"("error in (no error)"=w370, "Y axis value"=0.0, "X axis value"=w359, "RobotDriveDevRef"=w369) -> ()  [unwired: 5 in, 3 out]
          }
        }
        n263 = Greater?(x=w347, y=w346) -> (0:w345:bool)
        n264 = Wait (ms)(milliseconds to wait=u32 10) -> ()  [unwired: 1 out]
      }
    }
    frame Enabled {
    }
  }
